vi "AxAsyncLabVIEW.vi"() -> ()   [LabVIEW 2020, in "TrioMotion Controller.lvlib"]
uses:
  TrioMotion Controller.lvlib
panel:
  out "ModeChanged":bool
  out "CommPort":fxp<+,3,3>
  out "IsOpenLED":bool
  in  "Set Parameters":bool
  in  "Connection":string(combo)
  in  "Clear Windows":bool
  out "Responce (Channel 5)":string
  out "Responce (Normal/ Channel 0)":string
  in  "Commands (Normal/ Channel 0)":string
  in  "Send Commands":bool
  in  "Mode":enum32{"Radio Selection 1", "Radio Selection 2"}(radio)
  in  "Open/ Close":bool
  in  "stop":bool
  out "Error Out":errorcluster
  in  "Error In (no error)":errorcluster
  in  "Connection":refnum<k7>(container)
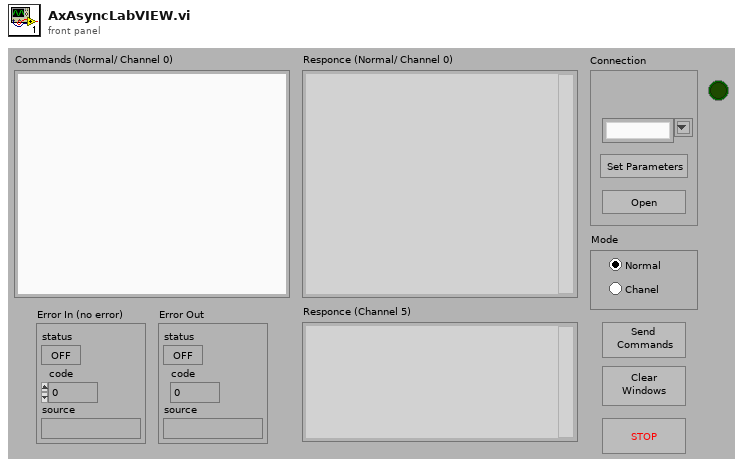
[diagram p1: front panel]
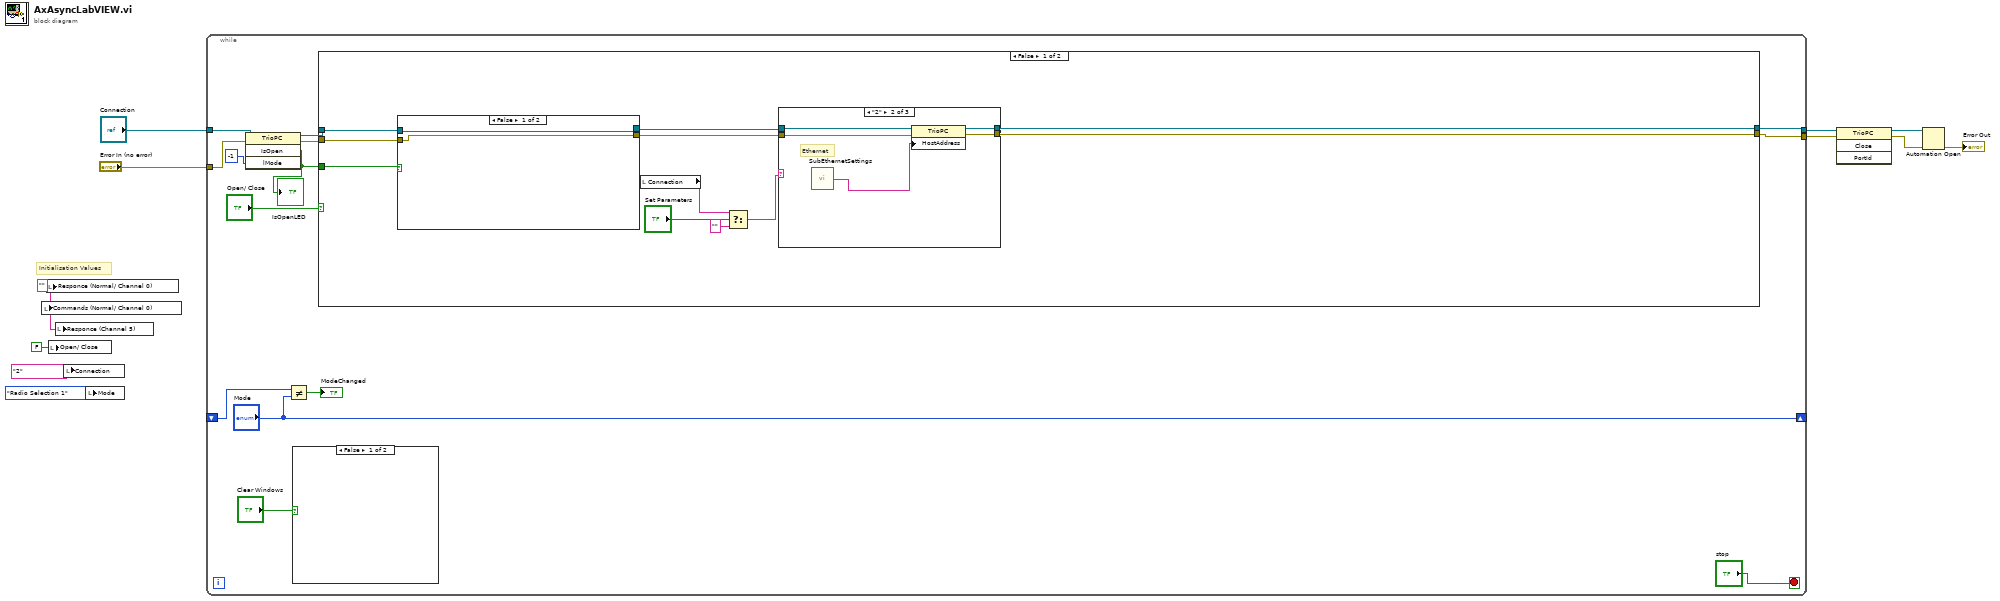
[diagram p0: block diagram]
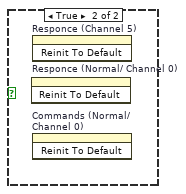
[diagram p2: hidden frame]
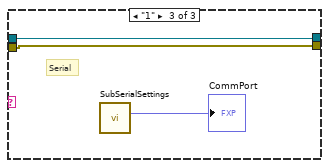
[diagram p4: hidden frame]
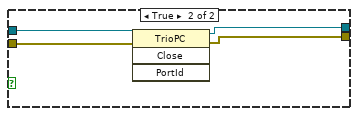
[diagram p5: hidden frame]
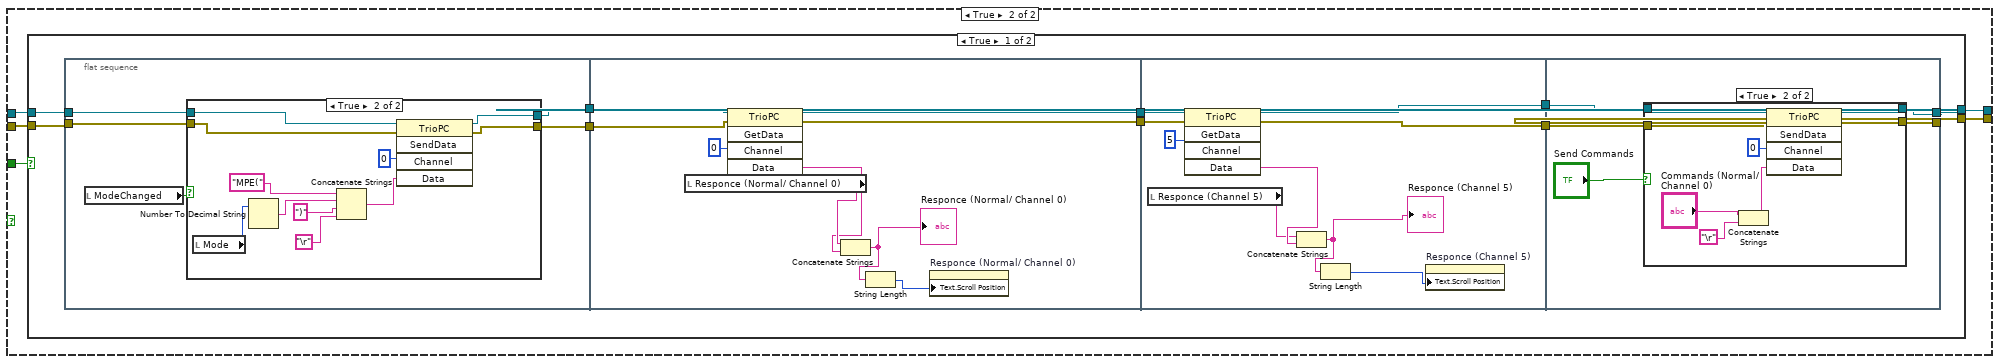
[diagram p6: hidden frame]
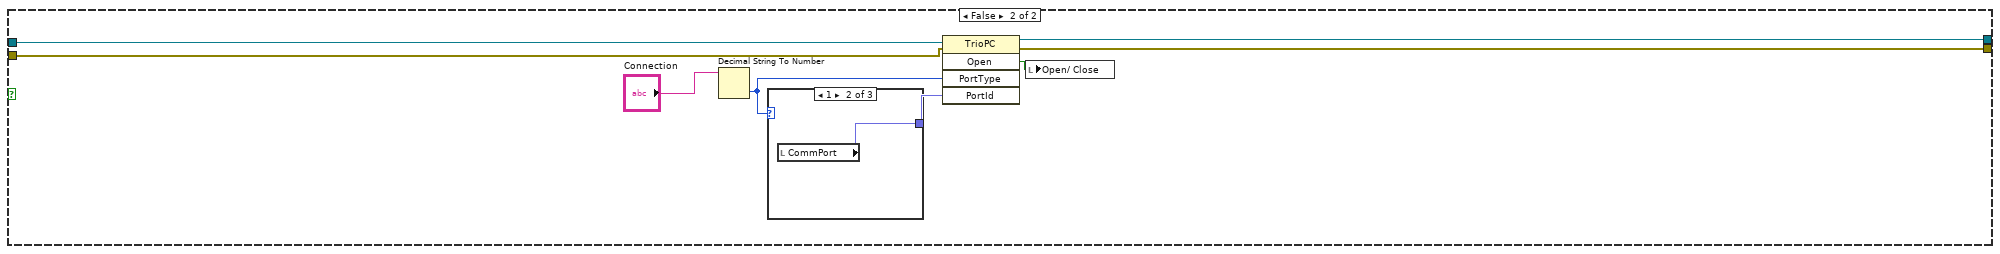
[diagram p9: hidden frame]
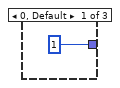
[diagram p10: hidden frame]
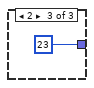
[diagram p11: hidden frame]
diagram:
  w3 = "" ("Responce (Normal/ Channel 0)")
  # "Initialisation Values"
  n1 = local write "Commands (Normal/ Channel 0)"(w3) -> ()
  n2 = local write "Responce (Normal/ Channel 0)"(w3) -> ()
  n3 = local write "Open/ Close"(FALSE ("Open/ Close")) -> ()
  n4 = local write "Responce (Channel 5)"(w3) -> ()
  n5 = local write "Connection"("2" ("Connection")) -> ()
  n6 = local write "Mode"(enum32{"Radio Selection 1", "Radio Selection 2"}."Radio Selection 1" ("Mode")) -> ()
  n7 = while {
    tunnel: "Connection" -> [w19]
    tunnel: [w24] -> w6
    tunnel: "Error In (no error)" -> [w18]
    tunnel: [w23] -> w5
    shift-right: ["Mode"] -> _
    shift-left: _ -> [w15]
    stop <- "stop" stop-if-true
    n8 = invoke class="TrioPC" method="IsOpen"(reference=w19, error in=w18, "lMode"=-1) -> (reference out=w21:refnum<k7>, error out=w20:errorcluster, "IsOpen"=w13:bool)  [unwired: 1 in, 1 out]
    "IsOpenLED" <- w13
    n9 = Not Equal?(x=w15, y="Mode") -> (x != y?=→"ModeChanged":bool)
    n10 = case shown="False" "Clear Windows" {
      frame False {
      }
      frame True {
        n11 = invoke on="Responce (Normal/ Channel 0)" class="Str" method="Reinit To Default"() -> ()  [unwired: 3 in, 3 out]
        n12 = invoke on="Responce (Channel 5)" class="Str" method="Reinit To Default"() -> ()  [unwired: 3 in, 3 out]
        n13 = invoke on="Commands (Normal/ Channel 0)" class="Str" method="Reinit To Default"() -> ()  [unwired: 3 in, 3 out]
      }
    }
    n14 = case shown="False" "Open/ Close" {
      tunnel: w21 -> [w36 w55]
      tunnel: w20 -> [w35 w54]
      tunnel: [w28 w57] -> w24
      tunnel: [w27 w56] -> w23
      tunnel: w13 -> [w34 w53]
      frame False {
        n15 = case shown="False" w34 {
          tunnel: w36 -> [w48 w52]
          tunnel: w35 -> [w47 w51]
          tunnel: [w48 w50] -> w30
          tunnel: [w47 w49] -> w29
          frame False {
          }
          frame True {
            n16 = invoke class="TrioPC" method="Close"(reference=w52, error in=w51) -> (reference out=w50:refnum<k7>, error out=w49:errorcluster)  [unwired: 2 in, 2 out]
          }
        }
        n17 = local read "Connection"() -> (w26:string)
        n18 = Select(t=w26, s="Set Parameters", f="") -> (s? t:f=w31:string)
        n19 = case shown="\"2\"" w31 {
          tunnel: w30 -> [w38 w41 w46]
          tunnel: w29 -> [w37 w40 w45]
          tunnel: [w38 w43 w46] -> w28
          tunnel: [w37 w42 w45] -> w27
          frame "", Default {
          }
          frame "2" {
            # "Ethernet"
            n20 = call "SubEthernetSettings.vi"() -> ("Ethernet IP Address 2"=w39:string)
            n21 = property class="TrioPC"(reference=w41, error in=w40, "HostAddress"=w39) -> (reference out=w43:refnum<k7>, error out=w42:errorcluster)
          }
          frame "1" {
            # "Serial"
            n22 = call "SubSerialSettings.vi"() -> ("CommPort"=→"CommPort":fxp<+,3,3>)
          }
        }
      }
      frame True {
        n23 = case shown="True" w53 {
          tunnel: w55 -> [w67 w124]
          tunnel: w54 -> [w66 w123]
          tunnel: [w65 w122] -> w57
          tunnel: [w64 w121] -> w56
          frame True {
            n24 = flat-sequence {
              tunnel: w67 -> [w71]
              tunnel: w66 -> [w70]
              tunnel: [w69] -> w63
              tunnel: [w68] -> w62
              tunnel: w63 -> [w93]
              tunnel: w62 -> [w90]
              tunnel: [w92] -> w61
              tunnel: [w91] -> w59
              tunnel: w61 -> [w101]
              tunnel: [w99] -> w60
              tunnel: w59 -> [w100]
              tunnel: [w98] -> w58
              tunnel: [w107] -> w65
              tunnel: [w106] -> w64
              tunnel: w60 -> [w108]
              tunnel: w58 -> [w105]
              frame #0 {
                n25 = local read "ModeChanged"() -> (w72:bool)
                n26 = case shown="True" w72 {
                  tunnel: w71 -> [w74 w85]
                  tunnel: w70 -> [w73 w84]
                  tunnel: [w74 w83] -> w69
                  tunnel: [w73 w82] -> w68
                  frame False {
                  }
                  frame True {
                    n27 = local read "Mode"() -> (w76:enum32{"Radio Selection 1", "Radio Selection 2"})
                    n28 = Number To Decimal String(number=w76) -> (decimal integer string=w79:string)  [unwired: 1 in]
                    n29 = Concatenate Strings("MPE(" ("Data"), w79, ")", "\r") -> (w77:string)
                    n30 = invoke class="TrioPC" method="SendData"(reference=w85, error in=w84, "Channel"=i16 0, "Data"=w77) -> (reference out=w83:refnum<k7>, error out=w82:errorcluster)  [unwired: 1 in, 3 out]
                  }
                }
              }
              frame #1 {
                n31 = local read "Responce (Normal/ Channel 0)"() -> (w89:string)
                n32 = invoke class="TrioPC" method="GetData"(reference=w93, error in=w90, "Channel"=i16 0) -> (reference out=w92:refnum<k7>, error out=w91:errorcluster, "Data"=w88:string)  [unwired: 2 in, 2 out]
                n33 = Concatenate Strings(w89, w88) -> (w86:string)
                "Responce (Normal/ Channel 0)" <- w86
                n34 = String Length(string=w86) -> (length=w87:i32)
                n35 = property on="Responce (Normal/ Channel 0)" class="Str"("Text.Scroll Position"=w87) -> ()  [unwired: 2 in, 2 out]
              }
              frame #2 {
                n36 = local read "Responce (Channel 5)"() -> (w95:string)
                n37 = invoke class="TrioPC" method="GetData"(reference=w101, error in=w100, "Channel"=i16 5) -> (reference out=w99:refnum<k7>, error out=w98:errorcluster, "Data"=w102:string)  [unwired: 2 in, 2 out]
                n38 = Concatenate Strings(w95, w102) -> (w97:string)
                "Responce (Channel 5)" <- w97
                n39 = String Length(string=w97) -> (length=w96:i32)
                n40 = property on="Responce (Channel 5)" class="Str"("Text.Scroll Position"=w96) -> ()  [unwired: 2 in, 2 out]
              }
              frame #3 {
                n41 = case shown="True" "Send Commands" {
                  tunnel: w108 -> [w109 w118]
                  tunnel: [w109 w117] -> w107
                  tunnel: [w110 w116] -> w106
                  tunnel: w105 -> [w110 w115]
                  frame False {
                  }
                  frame True {
                    n42 = Concatenate Strings("Commands (Normal/ Channel 0)", "\r") -> (w111:string)
                    n43 = invoke class="TrioPC" method="SendData"(reference=w118, error in=w115, "Channel"=i16 0, "Data"=w111) -> (reference out=w117:refnum<k7>, error out=w116:errorcluster)  [unwired: 1 in, 3 out]
                  }
                }
              }
            }
          }
          frame False {
            n44 = Decimal String To Number(string="Connection") -> (number=w125:i32)  [unwired: 2 in, 1 out]
            n45 = case shown="1" w125 {
              tunnel: [i16 1 ("PortId") w128 i16 23 ("PortId")] -> w126
              frame 0, Default {
              }
              frame 1 {
                n46 = local read "CommPort"() -> (w128:fxp<+,3,3>)
              }
              frame 2 {
              }
            }
            n47 = invoke class="TrioPC" method="Open"(reference=w124, error in=w123, "PortType"=w125, "PortId"=w126) -> (reference out=w122:refnum<k7>, error out=w121:errorcluster, "Open"=w120:bool)  [unwired: 1 in, 2 out]
            n48 = local write "Open/ Close"(w120) -> ()
          }
        }
      }
    }
  }
  n49 = invoke class="TrioPC" method="Close"(reference=w6, error in=w5) -> (reference out=w10:refnum<k7>, error out=w9:errorcluster)  [unwired: 2 in, 2 out]
  n50 = Automation Open(error in (no error)=w9, Automation Refnum=w10) -> (error out=→"Error Out":errorcluster)  [unwired: 2 in, 1 out]
